vi "Open Utility Motors.vi"(9 "CAN IDs":u8[](array[numeric])) -> ()   [LabVIEW 2018]
uses:
  <vilib>/Rock Robotics/WPI/ThirdParty/Phoenix-LabVIEW/Motor Controller/Controls/CTRE_Phoenix_MotorControl_NeutralMode.ctl
  <vilib>/Rock Robotics/SystemInterfaces/DIO/FPGA_DIOChannel.ctl
  <vilib>/Rock Robotics/WPI/Switch/WPI_SwitchOpenLimit.vi
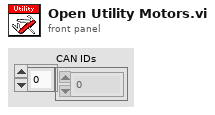
[diagram p1: front panel]
types:
  T1 = typedef "FPGA_DIOChannel.ctl" = enum8{"DIO 0", "DIO 1", "DIO 2", "DIO 3", "DIO 4", "DIO 5", "DIO 6", "DIO 7", "DIO 8", "DIO 9", "DIO MXP 0", "DIO MXP 1", "DIO MXP 2", "DIO MXP 3", "DIO MXP 4", "DIO MXP 5", "DIO MXP 6", "DIO MXP 7", "DIO MXP 8", "DIO MXP 9", "DIO MXP 10", "DIO MXP 11", "DIO MXP 12", "DIO MXP 13", "DIO MXP 14", "DIO MXP 15", "SPI Port CS1", "SPI Port CS2", "SPI Port CS3", "SPI Port MISO", "SPI Port MOSI", "Invalid"}
  T2 = typedef "CTRE_Phoenix_MotorControl_NeutralMode.ctl" = enum8{"EEPROMSetting", "Override to Coast", "Override to Brake"}
  T3 = typedef "WPI_MotorControlDeviceRef.ctl" = cluster{"DeviceStatus":errorcluster, "Type":T4, "PWM":cluster{"PWM Channel":T5, "DeadBand":T6}, "CAN":cluster{"Device Number":u8, "SetOutput VI Ref":variant, "GetOutput VI Ref":variant, "Enable VI Ref":variant, "Disable VI Ref":variant, "Data":variant}, "Invert":bool, "DIO PWM":cluster{"PWM \"Enable\" Channel":T5, "DIOChannel":T1, "PWM Rate":dbl}}
  T4 = typedef "WPI_MotorControlType.ctl" = enum16{"PWM", "CAN", "DIO PWM"}
  T5 = typedef "FPGA_DIOPWMChannel.ctl" = enum8{"PWM 0", "PWM 1", "PWM 2", "PWM 3", "PWM 4", "PWM 5", "PWM 6", "PWM 7", "PWM 8", "PWM 9", "PWM MXP 0", "PWM MXP 1", "PWM MXP 2", "PWM MXP 3", "PWM MXP 4", "PWM MXP 5", "PWM MXP 6", "PWM MXP 7", "PWM MXP 8", "PWM MXP 9", "Invalid"}
  T6 = typedef "WPI_PWMDeadband.ctl" = cluster{"Name":string, "maxPositivePwm":i32, "minPositivePwm":i32, "centerPwm":i32, "maxNegativePwm":i32, "minNegativePwm":i32, "angularRange":u16}
  T7 = typedef "WPI_SwitchDevRef.ctl" = cluster{"DevStatus":errorcluster, "DIO Channel":T1, "CntIndex":T8, "Normally Closed":bool}
  T8 = typedef "FPGA_CounterCtrSystemIndex.ctl" = enum8{"Ctr 0", "Ctr 1", "Ctr 2", "Ctr 3", "Ctr 4", "Ctr 5", "Ctr 6", "Ctr 7", "Invalid"}
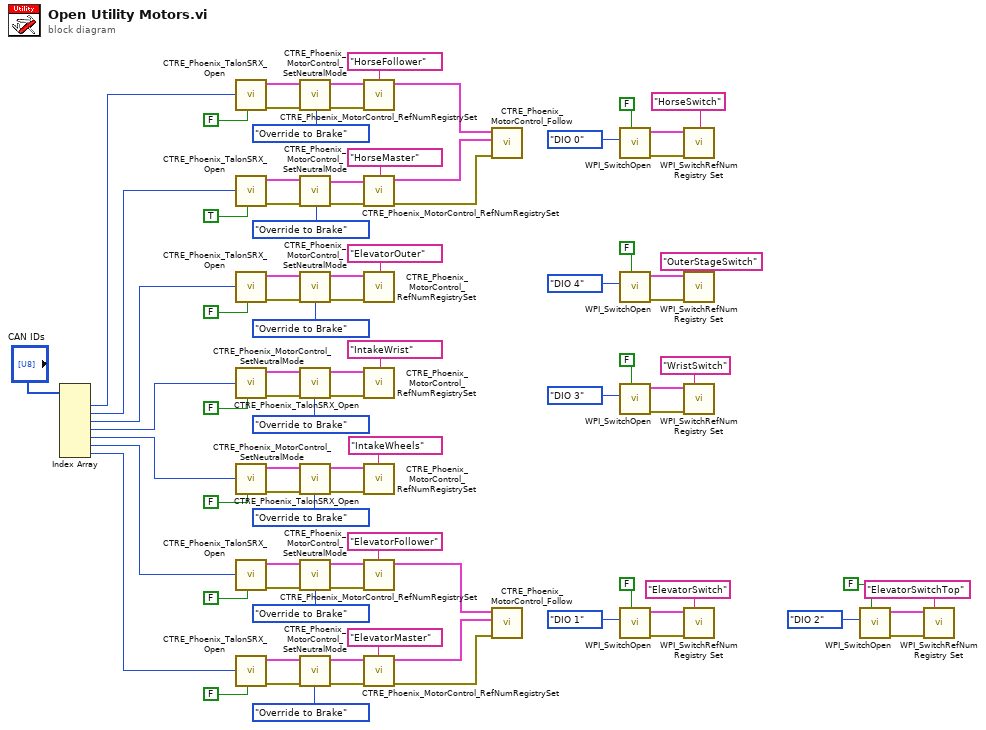
[diagram p0: block diagram]
diagram:
  n1 = Index Array(array="CAN IDs") -> (element #1=w39:u8, element #2=w38:u8, element #3=w37:u8, element #4=w36:u8, element #5=w35:u8, element #6=w34:u8, element #7=w33:u8)  [unwired: 7 in]
  n2 = call <vilib>:"CTRE_Phoenix_TalonSRX_Open.vi"("Invert"=FALSE, "Device Number"=w39) -> ("error out"=w88:errorcluster, "CAN Talon SRX Ref"=w74:T3)  [unwired: 8 in]
  n3 = call <vilib>:"CTRE_Phoenix_TalonSRX_Open.vi"("Invert"=TRUE, "Device Number"=w38) -> ("error out"=w86:errorcluster, "CAN Talon SRX Ref"=w72:T3)  [unwired: 8 in]
  n4 = call <vilib>:"CTRE_Phoenix_TalonSRX_Open.vi"("Invert"=FALSE, "Device Number"=w37) -> ("error out"=w84:errorcluster, "CAN Talon SRX Ref"=w70:T3)  [unwired: 8 in]
  n5 = call <vilib>:"CTRE_Phoenix_TalonSRX_Open.vi"("Invert"=FALSE, "Device Number"=w36) -> ("error out"=w82:errorcluster, "CAN Talon SRX Ref"=w68:T3)  [unwired: 8 in]
  n6 = call <vilib>:"CTRE_Phoenix_TalonSRX_Open.vi"("Invert"=FALSE, "Device Number"=w35) -> ("error out"=w80:errorcluster, "CAN Talon SRX Ref"=w66:T3)  [unwired: 8 in]
  n7 = call <vilib>:"CTRE_Phoenix_TalonSRX_Open.vi"("Invert"=FALSE, "Device Number"=w34) -> ("error out"=w78:errorcluster, "CAN Talon SRX Ref"=w64:T3)  [unwired: 8 in]
  n8 = call <vilib>:"CTRE_Phoenix_TalonSRX_Open.vi"("Invert"=FALSE, "Device Number"=w33) -> ("error out"=w76:errorcluster, "CAN Talon SRX Ref"=w62:T3)  [unwired: 8 in]
  n9 = call <vilib>:"CTRE_Phoenix_MotorControl_SetNeutralMode.vi"("error in (no error)"=w88, "Motor Control Neutral Mode"=CTRE_Phoenix_MotorControl_NeutralMode."Override to Brake", "PhoenixMotorControlDevRef"=w74) -> ("error out"=w87:errorcluster, "PhoenixMotorControlDevRef"=w73:T3)  [unwired: 7 in]
  n10 = call <vilib>:"CTRE_Phoenix_MotorControl_SetNeutralMode.vi"("error in (no error)"=w86, "Motor Control Neutral Mode"=CTRE_Phoenix_MotorControl_NeutralMode."Override to Brake", "PhoenixMotorControlDevRef"=w72) -> ("error out"=w85:errorcluster, "PhoenixMotorControlDevRef"=w71:T3)  [unwired: 7 in]
  n11 = call <vilib>:"CTRE_Phoenix_MotorControl_SetNeutralMode.vi"("error in (no error)"=w84, "Motor Control Neutral Mode"=CTRE_Phoenix_MotorControl_NeutralMode."Override to Brake", "PhoenixMotorControlDevRef"=w70) -> ("error out"=w83:errorcluster, "PhoenixMotorControlDevRef"=w69:T3)  [unwired: 7 in]
  n12 = call <vilib>:"CTRE_Phoenix_MotorControl_SetNeutralMode.vi"("error in (no error)"=w82, "Motor Control Neutral Mode"=CTRE_Phoenix_MotorControl_NeutralMode."Override to Brake", "PhoenixMotorControlDevRef"=w68) -> ("error out"=w81:errorcluster, "PhoenixMotorControlDevRef"=w67:T3)  [unwired: 7 in]
  n13 = call <vilib>:"CTRE_Phoenix_MotorControl_SetNeutralMode.vi"("error in (no error)"=w80, "Motor Control Neutral Mode"=CTRE_Phoenix_MotorControl_NeutralMode."Override to Brake", "PhoenixMotorControlDevRef"=w66) -> ("error out"=w79:errorcluster, "PhoenixMotorControlDevRef"=w65:T3)  [unwired: 7 in]
  n14 = call <vilib>:"CTRE_Phoenix_MotorControl_SetNeutralMode.vi"("error in (no error)"=w78, "Motor Control Neutral Mode"=CTRE_Phoenix_MotorControl_NeutralMode."Override to Brake", "PhoenixMotorControlDevRef"=w64) -> ("error out"=w77:errorcluster, "PhoenixMotorControlDevRef"=w63:T3)  [unwired: 7 in]
  n15 = call <vilib>:"CTRE_Phoenix_MotorControl_SetNeutralMode.vi"("error in (no error)"=w76, "Motor Control Neutral Mode"=CTRE_Phoenix_MotorControl_NeutralMode."Override to Brake", "PhoenixMotorControlDevRef"=w62) -> ("error out"=w75:errorcluster, "PhoenixMotorControlDevRef"=w61:T3)  [unwired: 7 in]
  n16 = call <vilib>:"CTRE_Phoenix_MotorControl_RefNumRegistrySet.vi"("error in (no error)"=w87, "refnum name"="HorseFollower", "PhoenixMotorControlDevRef"=w73) -> ("PhoenixMotorControlDevRef"=w31:T3)  [unwired: 7 in, 1 out]
  n17 = call <vilib>:"CTRE_Phoenix_MotorControl_RefNumRegistrySet.vi"("error in (no error)"=w85, "refnum name"="HorseMaster", "PhoenixMotorControlDevRef"=w71) -> ("error out"=w29:errorcluster, "PhoenixMotorControlDevRef"=w30:T3)  [unwired: 7 in]
  n18 = call <vilib>:"CTRE_Phoenix_MotorControl_RefNumRegistrySet.vi"("error in (no error)"=w83, "refnum name"="ElevatorOuter", "PhoenixMotorControlDevRef"=w69) -> ()  [unwired: 7 in, 2 out]
  n19 = call <vilib>:"CTRE_Phoenix_MotorControl_RefNumRegistrySet.vi"("error in (no error)"=w81, "refnum name"="IntakeWrist", "PhoenixMotorControlDevRef"=w67) -> ()  [unwired: 7 in, 2 out]
  n20 = call <vilib>:"CTRE_Phoenix_MotorControl_RefNumRegistrySet.vi"("error in (no error)"=w79, "refnum name"="IntakeWheels", "PhoenixMotorControlDevRef"=w65) -> ()  [unwired: 7 in, 2 out]
  n21 = call <vilib>:"CTRE_Phoenix_MotorControl_RefNumRegistrySet.vi"("error in (no error)"=w77, "refnum name"="ElevatorFollower", "PhoenixMotorControlDevRef"=w63) -> ("PhoenixMotorControlDevRef"=w28:T3)  [unwired: 7 in, 1 out]
  n22 = call <vilib>:"CTRE_Phoenix_MotorControl_RefNumRegistrySet.vi"("error in (no error)"=w75, "refnum name"="ElevatorMaster", "PhoenixMotorControlDevRef"=w61) -> ("error out"=w26:errorcluster, "PhoenixMotorControlDevRef"=w27:T3)  [unwired: 7 in]
  n23 = call <vilib>:"CTRE_Phoenix_MotorControl_Follow.vi"("error in (no error)"=w29, "Master Controller to Follow"=w30, "PhoenixMotorControlDevRef"=w31) -> ()  [unwired: 7 in, 2 out]
  n24 = call <vilib>:"CTRE_Phoenix_MotorControl_Follow.vi"("error in (no error)"=w26, "Master Controller to Follow"=w27, "PhoenixMotorControlDevRef"=w28) -> ()  [unwired: 7 in, 2 out]
  n25 = call-poly <vilib>:"WPI_SwitchOpen.vi"("Normally Closed"=FALSE, "DIO Channel"=FPGA_DIOChannel."DIO 0") -> ("error out"=w24:errorcluster, "SwitchDevRef"=w25:T7)  [unwired: 8 in]
  n26 = call-poly <vilib>:"WPI_SwitchOpen.vi"("Normally Closed"=FALSE, "DIO Channel"=FPGA_DIOChannel."DIO 4") -> ("error out"=w4:errorcluster, "SwitchDevRef"=w3:T7)  [unwired: 8 in]
  n27 = call-poly <vilib>:"WPI_SwitchOpen.vi"("Normally Closed"=FALSE, "DIO Channel"=FPGA_DIOChannel."DIO 3") -> ("error out"=w7:errorcluster, "SwitchDevRef"=w8:T7)  [unwired: 8 in]
  n28 = call-poly <vilib>:"WPI_SwitchOpen.vi"("Normally Closed"=FALSE, "DIO Channel"=FPGA_DIOChannel."DIO 1") -> ("error out"=w21:errorcluster, "SwitchDevRef"=w20:T7)  [unwired: 8 in]
  n29 = call <vilib>:"WPI_SwitchRefNum Registry Set.vi"("error in (no error)"=w24, "refnum name"="HorseSwitch", "SwitchDevRef"=w25) -> ()  [unwired: 7 in, 2 out]
  n30 = call <vilib>:"WPI_SwitchRefNum Registry Set.vi"("error in (no error)"=w4, "refnum name"="OuterStageSwitch", "SwitchDevRef"=w3) -> ()  [unwired: 7 in, 2 out]
  n31 = call <vilib>:"WPI_SwitchRefNum Registry Set.vi"("error in (no error)"=w7, "refnum name"="WristSwitch", "SwitchDevRef"=w8) -> ()  [unwired: 7 in, 2 out]
  n32 = call <vilib>:"WPI_SwitchRefNum Registry Set.vi"("error in (no error)"=w21, "refnum name"="ElevatorSwitch", "SwitchDevRef"=w20) -> ()  [unwired: 7 in, 2 out]
  n33 = call-poly <vilib>:"WPI_SwitchOpen.vi"("Normally Closed"=FALSE, "DIO Channel"=FPGA_DIOChannel."DIO 2") -> ("error out"=w12:errorcluster, "SwitchDevRef"=w13:T7)  [unwired: 8 in]
  n34 = call <vilib>:"WPI_SwitchRefNum Registry Set.vi"("error in (no error)"=w12, "refnum name"="ElevatorSwitchTop", "SwitchDevRef"=w13) -> ()  [unwired: 7 in, 2 out]
